vi "PUT (Buffer).vi"(6 "timeout":i32=10000, 7 "output file":path, 8 "error in":errorcluster, 9 "buffer":string, 10 "url":string, 11 "http-method in":refnum<class "http-client.lvclass">) -> (0 "error out":errorcluster, 2 "response":refnum<class "response.lvclass">, 3 "http-method out":refnum<class "http-client.lvclass">)   [LabVIEW 2020, in "http.lvlib" / "http-client.lvclass"]
uses:
  http-client.lvclass
  response/response.lvclass
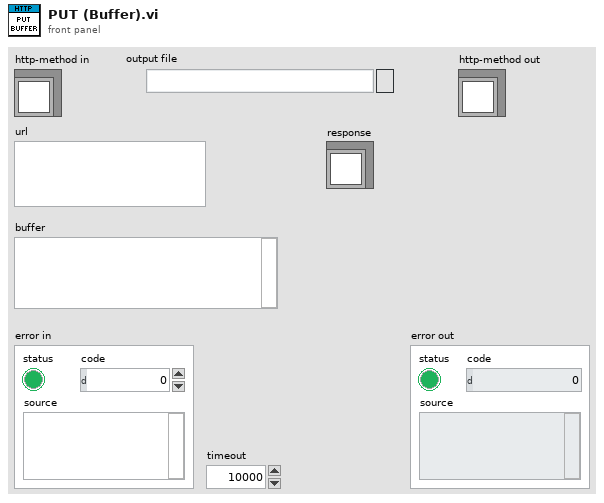
[diagram p1: front panel]
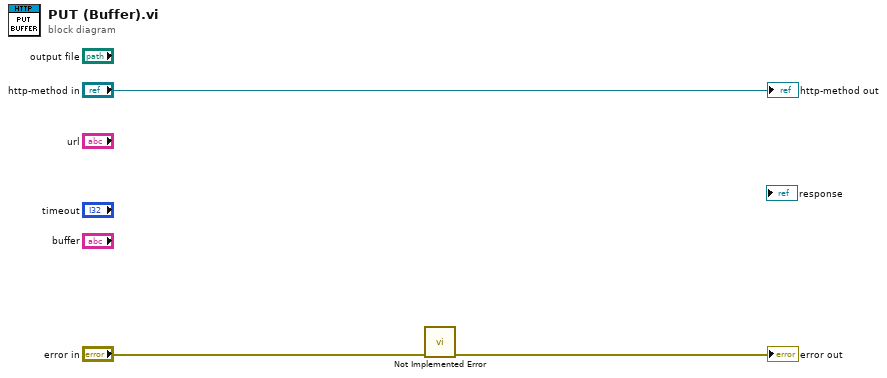
[diagram p0: block diagram]
diagram:
  n1 = call "Not Implemented Error.vi"("error in (no error)"="error in") -> ("error out"=→"error out":errorcluster)  [unwired: 10 in]
  "http-method out" <- "http-method in"
